vi "Power & Frequency Estimator.vi"() -> ()   [LabVIEW 2023]
doc: "Demonstrates how to use the Power & Frequency Estimate VI to estimate the peak of a signal. This technique is useful when the real peak does not occur at the exact frequency bin in the power spectrum or when the window is used."
uses:
  <vilib>/Analysis/1siggen.llb/Ramp Pattern by Samples.vi
  <vilib>/Analysis/0measdsp.llb/Scaled Time Domain Window (DBL).vi
  <vilib>/measure/NI_MABase.lvlib
  <vilib>/Analysis/NI_AALPro.lvlib
  <vilib>/Analysis/NI_AALBase.lvlib
panel:
  in  "window":u32(ring)=1 items=["Rectangle"=0, "Hanning"=1, "Hamming"=2, "Blackman-Harris"=3, "Exact Blackman"=4, "Blackman"=5, "Flat Top"=6, "4 Term B-Harris "=7, "7 Term B-Harris"=8, "Low Sidelobe"=9, "Blackman Nuttall"=11, "Triangle"=30, "Bartlett-Hanning"=31, "Bohman"=32, "Parzen"=33, "Welch"=34, "Kaiser"=60, "Dolph-Chebyshev"=61, "Gaussian"=62]
  in  "span (bins)":i32=7 format="%0.0f"
  out "Time-Domain Signal":waveform(dbl)(graph)
  in  "Input Signal":T1(array[cluster])=[{"frequency (Hz)"=12.7, "amplitude"=1.0, "phase"=0.0}, {"frequency (Hz)"=21.5, "amplitude"=0.8, "phase"=0.0}]
  out "Power Spectrum":T2(graph)
  out "Estimated Frequency Peak (hz)":dbl[](array[numeric])
  out "Estimated Power Peak":dbl[](array[numeric])
  # "Overview: This example shows how to use the Power & Frequency Estimate VI to estimate the peak frequency and power in a power spectrum.\nRequirements: LabVIEW Full Development System\nInstructions: \n1. Run the VI and note that the Estimated Frequency Peak and Estimated Power Peak values are close to the expected theoretical values.\n2. Change the Input Signal and span, then run the VI to see the new Power Spectrum and estimated frequency and power peak values."
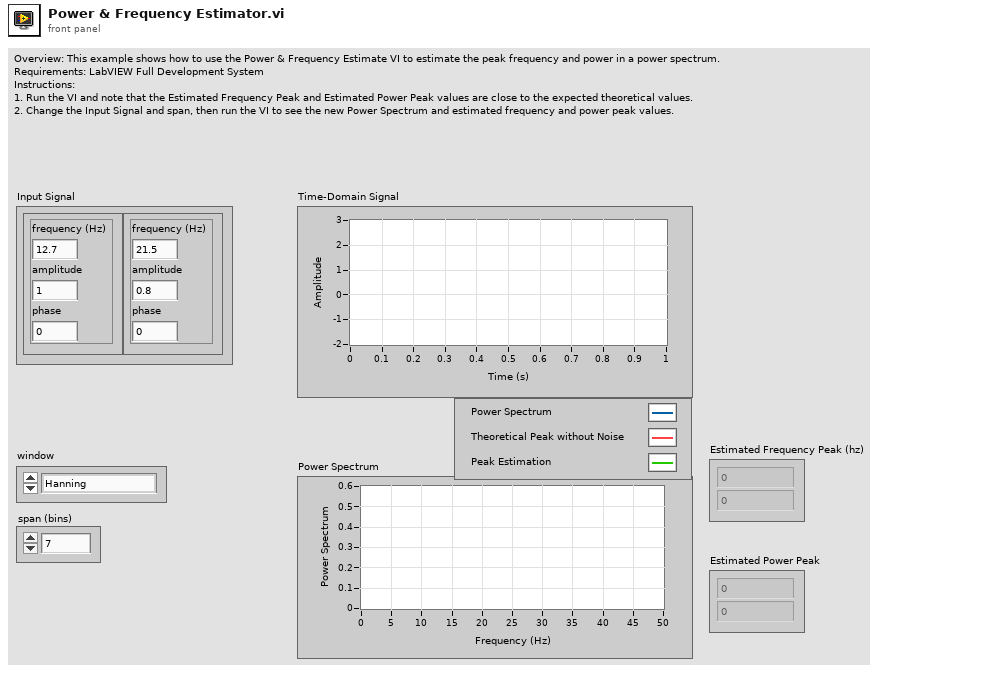
[diagram p1: front panel]
types:
  T1 = cluster{"frequency (Hz)":dbl, "amplitude":dbl, "phase":dbl}[]
  T2 = cluster{dbl[], "Power Spectrum (V^2 rms)":dbl[]}[]
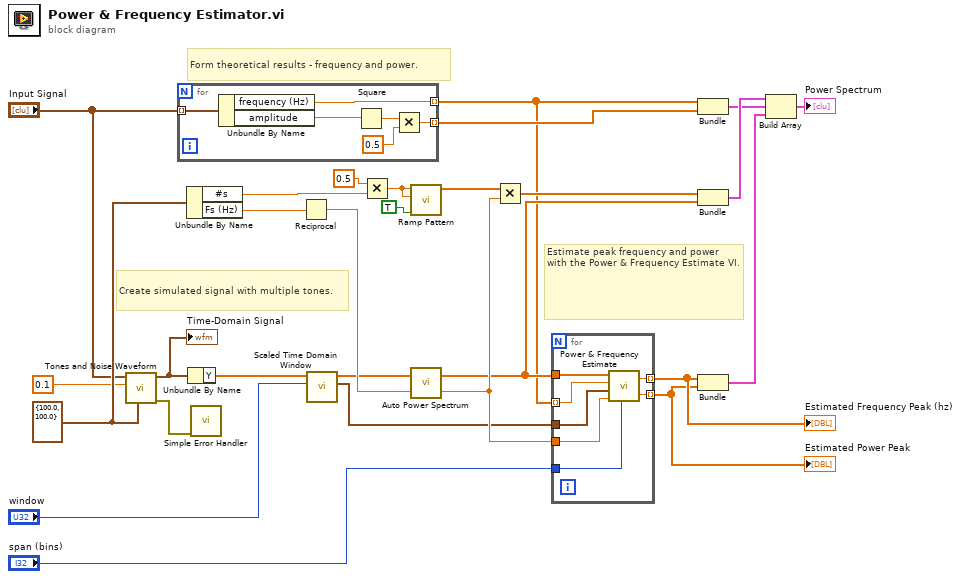
[diagram p0: block diagram]
diagram:
  w26 = cluster{"Fs (Hz)":dbl, "#s":dbl} {"Fs (Hz)"=100.0, "#s"=100.0} ("sampling info")
  # "Create simulated signal with multiple tones."
  # "Estimate peak frequency and power with the Power & Frequency Estimate VI."
  # "Form theoretical results - frequency and power."
  n1 = call <vilib>:"Tones and Noise Waveform.vi"("sampling info"=w26, "noise (rms)"=0.1, "tones"="Input Signal") -> ("error out"=w1:errorcluster, "signal out"=w24:waveform(dbl))  [unwired: 7 in]
  "Time-Domain Signal" <- w24
  n2 = for {
    tunnel: "Input Signal" -> [w34] mode=indexing
    tunnel: [w33] -> w3 mode=indexing
    tunnel: [w29] -> w13 mode=indexing
    n3 = Unbundle By Name(w34) -> ("frequency (Hz)"=w33:dbl, "amplitude"=w32:dbl)
    n4 = Square(x=w32) -> (x^2=w31:dbl)
    n5 = Multiply(x=w31, y=0.5) -> (x*y=w29:dbl)
  }
  n6 = Unbundle By Name(w26) -> ("#s"=w7:dbl, "Fs (Hz)"=w8:dbl)
  n7 = Unbundle By Name(w24) -> ("Y"=w12:dbl[])
  n8 = call <vilib>:"Simple Error Handler.vi"("error in (no error)"=w1) -> ()  [unwired: 4 in, 5 out]
  n9 = Reciprocal(x=w8) -> (1/x=w25:dbl)
  n10 = call-poly <vilib>:"Scaled Time Domain Window.vi"("window"="window", "X"=w12) -> ("window properties"=w10:cluster{"eq noise BW":dbl, "coherent gain":dbl}, "Windowed X"=w11:dbl[])  [unwired: 7 in, 1 out]
  n11 = Multiply(x=0.5 ("y"), y=w7) -> (x*y=w28:dbl)
  n12 = call-poly <vilib>:"Ramp Pattern.vi"("exclude end?"=TRUE, "end"=w28, "samples"=w28) -> ("Ramp Pattern"=w17:dbl[])  [unwired: 7 in, 1 out]
  n13 = call <vilib>:"Auto Power Spectrum.vi"("dt"=w25, "Signal (V)"=w11) -> ("df"=w27:dbl, "Power Spectrum (V^2 rms)"=w22:dbl[])
  n14 = Multiply(x=w17, y=w27) -> (x*y=w16:dbl[])
  n15 = for {
    tunnel: w22 -> [w41]
    tunnel: w27 -> [w40]
    tunnel: [w39] -> w20 mode=indexing
    tunnel: [w38] -> w19 mode=indexing
    tunnel: w3 -> [w37] mode=indexing
    tunnel: "span (bins)" -> [w36]
    tunnel: w10 -> [w35]
    n16 = call <vilib>:"Power & Frequency Estimate.vi"("span"=w36, "df"=w40, "window constants"=w35, "peak frequency (max)"=w37, "Power Spectrum (V^2 rms)"=w41) -> ("est power peak"=w38:dbl, "est frequency peak"=w39:dbl)  [unwired: 1 in]
  }
  "Estimated Power Peak" <- w19
  "Estimated Frequency Peak (hz)" <- w20
  n17 = Bundle(w3, w13) -> (w5:cluster{dbl[], dbl[]})  [unwired: 1 in]
  n18 = Bundle(w16, "Power Spectrum (V^2 rms)"=w22) -> (w6:cluster{dbl[], "Power Spectrum (V^2 rms)":dbl[]})  [unwired: 1 in]
  n19 = Bundle(w20, w19) -> (w9:cluster{dbl[], dbl[]})  [unwired: 1 in]
  n20 = Build Array(w6, w5, w9) -> (→"Power Spectrum":T2)
